vi "CFTS-Read State.vi"(0 "State In":T1, 11 "error in (no error)":errorcluster) -> (4 "State Out":T1, 15 "error out":errorcluster)   [LabVIEW 2020]
uses:
  CFTS-Experiment State.ctl
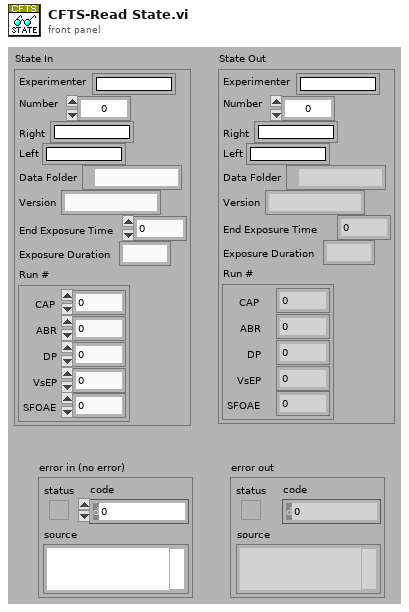
[diagram p1: front panel]
types:
  T1 = typedef "CFTS-Experiment State.ctl" = cluster{"Experimenter":string, "Number":u32, "Right":string, "Left":string, "Data Folder":path, "Version":string, "End Exposure Time":dbl, "Exposure Duration":string, "Run #":cluster{"CAP":i32, "ABR":i32, "DP":i32, "VsEP":i32, "SFOAE":i32}}
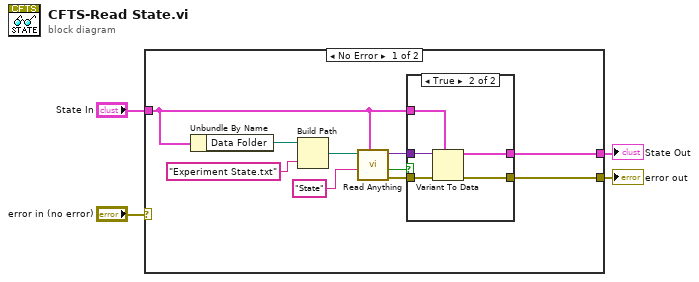
[diagram p0: block diagram]
diagram:
  n1 = case shown="No Error" "error in (no error)" {
    selector: "error in (no error)" -> [_ w22]
    tunnel: [w7 w22] -> w4
    tunnel: [w8 w23] -> w1
    tunnel: "State In" -> [w9 w23]
    frame No Error {
      n2 = Unbundle By Name(w9) -> ("Data Folder"=w14:path)
      n3 = Build Path(base path=w14, name or relative path="Experiment State.txt") -> (appended path=w12:path)
      n4 = call "Read Anything.vi"("Type of Anything"=w9, "Section Name (Name of \"Type of Anything\")"="State" ("Section Name (Name of \"Type of Anything\")"), "Path (dialog)"=w12) -> ("Error Out"=w11:errorcluster, "Found?"=w10:bool, "Anything"=w6:variant)  [unwired: 6 in]
      n5 = case shown="True" w10 {
        tunnel: w11 -> [w15 w21]
        tunnel: w9 -> [w16 w20]
        tunnel: [w16 w19] -> w8
        tunnel: [w15 w18] -> w7
        tunnel: w6 -> [_ w17]
        frame False {
        }
        frame True {
          n6 = Variant To Data(error in=w21, type=w20, Variant=w17) -> (data=w19:T1, error out=w18:errorcluster)
        }
      }
    }
    frame Error {
    }
  }
  "error out" <- w4
  "State Out" <- w1
